vi "NXT Move the tug A.vi"(0 "Arbiter Heading":i16 step=10, 1 "Desired Speed":i16 step=10) -> (2 "Right turn?":bool, 3 "Rudder":u16, 4 "Motor":u16)   [LabVIEW 2012, in "ENGR3390 Tug Boat.lvrbt"]
doc: "This is the VI NXT module for moving the tug. It accepts present and desired heading in degrees and desired motor speed and presents rudder and motor values and a right turn indicator."
uses:
  <vilib>/NXT/Dual Mode Library/prims/notExclusiveOr.vi
  <vilib>/NXT/Dual Mode Library/prims/inRangeAndCoerce/inRangeAndCoerce_int.vi
  ENGR3390 Tug Boat.lvrbt
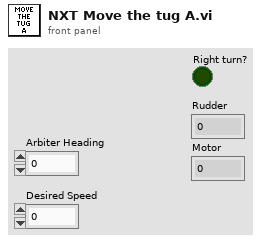
[diagram p1: front panel]
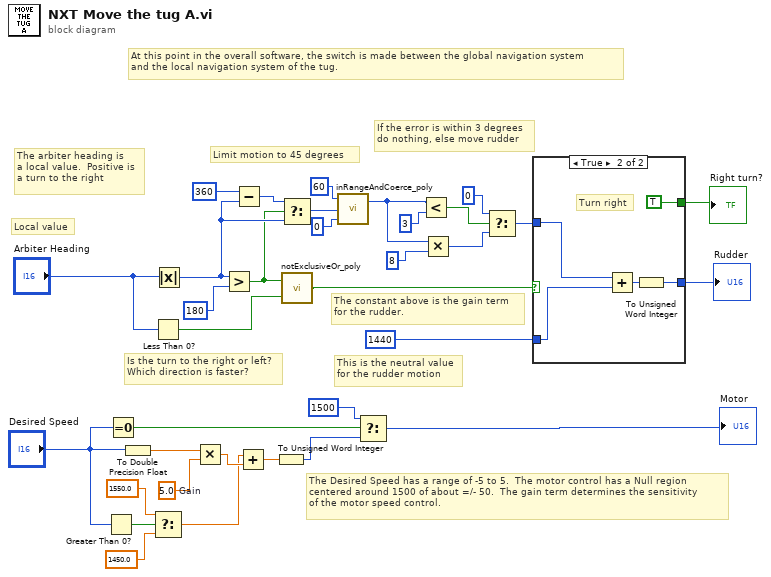
[diagram p0: block diagram]
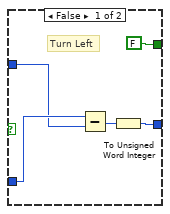
[diagram p2: hidden frame]
diagram:
  w28 = 5.0  # Gain
  # "The Desired Speed has a range of -5 to 5.  The motor control has a Null region\ncentered around 1500 of about =/- 50.  The gain term determines the sensitivity\nof the motor speed control."
  # "This is the neutral value\nfor the rudder motion"
  # "If the error is within 3 degrees\ndo nothing, else move rudder"
  # "The constant above is the gain term\nfor the rudder."
  # "The arbiter heading is \na local value.  Positive is\na turn to the right"
  # "Local value"
  # "At this point in the overall software, the switch is made between the global navigation system\nand the local navigation system of the tug."
  # "Limit motion to 45 degrees"
  # "Is the turn to the right or left?\nWhich direction is faster?"
  n1 = Greater Than 0?(x="Desired Speed") -> (x > 0?=w4:bool)
  n2 = Equal To 0?(x="Desired Speed") -> (x = 0?=w9:bool)
  n3 = To Double Precision Float(number="Desired Speed") -> (double precision float=w24:dbl)
  n4 = Less Than 0?(x="Arbiter Heading") -> (x < 0?=w22:bool)
  n5 = Select(t=1550.0, s=w4, f=1450.0) -> (s? t:f=w1:dbl)
  n6 = Absolute Value(x="Arbiter Heading") -> (abs(x)=w30:i16)
  n7 = Multiply(x=w24, y=w28) -> (x*y=w20:dbl)
  n8 = Greater?(x=w30, y=i16 180) -> (0:w23:bool)
  n9 = Subtract(x=i16 360, y=w30) -> (x-y=w29:i16)
  n10 = Add(x=w1, y=w20) -> (x+y=w10:dbl)
  n11 = To Unsigned Word Integer(number=w10) -> (unsigned 16bit integer=w7:u16)
  n12 = Select ("Absolute\nheading \nchange")(t=w29, s=w23, f=w30) -> (s? t:f=w27:i16)
  n13 = call-poly <vilib>:"notExclusiveOr_poly.vi"("y"=w22, "x"=w23) -> (".not. (x xor. y)?"=w21:bool)
  n14 = call-poly <vilib>:"inRangeAndCoerce_poly.vi"("lower limit"=0, "x"=w27, "upper limit"=60) -> ("coerced(x)"=w13:i32)  [unwired: 1 out]
  n15 = Select(t=u16 1500, s=w9, f=w7) -> (s? t:f=→"Motor":u16)
  n16 = Less?(x=w13, y=3) -> (x < y?=w16:bool)
  n17 = Multiply(x=w13, y=8) -> (x*y=w15:i32)
  n18 = Select(t=0, s=w16, f=w15) -> (s? t:f=w11:i32)
  n19 = case shown="True" w21 {
    tunnel: [w38 w42] -> w34
    tunnel: [FALSE TRUE] -> w33
    tunnel: 1440 -> [w36 w41]
    tunnel: w11 -> [w35 w40]
    frame False {
      # "Turn Left"
      n20 = Subtract(x=w36, y=w35) -> (x-y=w37:i32)
      n21 = To Unsigned Word Integer(number=w37) -> (unsigned 16bit integer=w38:u16)
    }
    frame True {
      # "Turn right"
      n22 = Add(x=w40, y=w41) -> (x+y=w43:i32)
      n23 = To Unsigned Word Integer(number=w43) -> (unsigned 16bit integer=w42:u16)
    }
  }
  "Rudder" <- w34
  "Right turn?" <- w33
